vi "Add State Callback.vi"(7 "Owner":refnum<class>, 8 "error in (no error)":errorcluster, 10 "Callback":refnum<vi>, 11 "Connection in":refnum<class "Connection.lvclass">) -> (0 "error out":errorcluster, 3 "Connection out":refnum<class "Connection.lvclass">)   [LabVIEW 2012, in "Stream.lvlib" / "Connection.lvclass"]
uses:
  Connection.lvclass
  Endpoint/Endpoint.lvclass
  Connection State.ctl
  Stream.lvlib
  Endpoint/State Callback.ctl
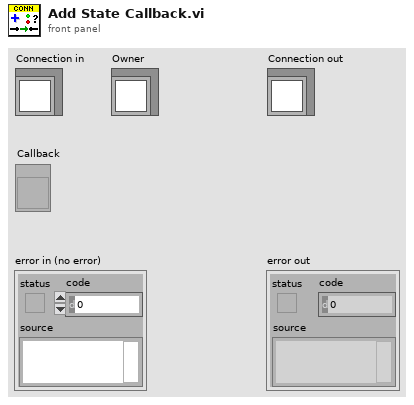
[diagram p1: front panel]
types:
  T1 = typedef "Stream.lvlib/Endpoint.lvclass/State Callback.ctl" = cluster{"Owner":refnum<class>, "VI":refnum<vi>}
  T2 = typedef "Stream.lvlib/Connection State.ctl" = enum16{"Connected", "Disconnected"}
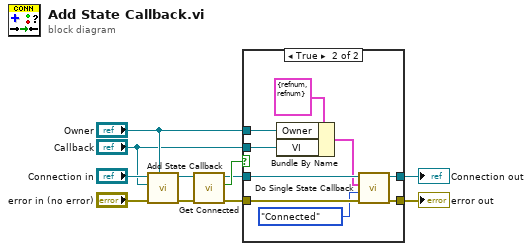
[diagram p0: block diagram]
diagram:
  n1 = call-parent "Add State Callback.vi"("Owner"="Owner", "error in (no error)"="error in (no error)", "Callback"="Callback", "Endpoint in"="Connection in") -> ("error out"=w8:errorcluster, "Endpoint out"=w9:refnum<class "Connection.lvclass">)  [unwired: 6 in]
  n2 = call-dynamic "Get Connected.vi"("error in (no error)"=w8, "Connection in"=w9) -> ("error out"=w5:errorcluster, "Connected"=w7:bool, "Connection out"=w6:refnum<class "Connection.lvclass">)  [unwired: 7 in]
  n3 = case shown="True" w7 {
    tunnel: w6 -> [w13 w21]
    tunnel: w5 -> [w12 w22]
    tunnel: [w13 w20] -> w4
    tunnel: [w12 w19] -> w3
    tunnel: "Owner" -> [_ w16]
    tunnel: "Callback" -> [_ w15]
    frame False {
    }
    frame True {
      n4 = Bundle By Name(cluster=T1 {"Owner"=refnum, "VI"=refnum} ("State Callback"), "Owner"=w16, "VI"=w15) -> (w14:T1)
      n5 = call "Do Single State Callback.vi"("error in (no error)"=w22, "State"=Connection_State."Connected", "State Callback"=w14, "Connection in"=w21) -> ("error out"=w19:errorcluster, "Connection out"=w20:refnum<class "Connection.lvclass">)  [unwired: 6 in]
    }
  }
  "error out" <- w3
  "Connection out" <- w4
